vi "Keyence.FTP.GetLastFile.vi"(5 "Bank (0)":u8, 7 "LogPath":path=path "C:/SOFTWARE/logs/scanner", 8 "error in (no error)":errorcluster, 11 "FTP Session out":T1) -> (0 "error out":errorcluster, 3 "File name":path)   [LabVIEW 2016]
uses:
  <vilib>/FTP/ftp0.llb/FTP Session.ctl
  <vilib>/FTP/NI_FTP.lvlib
panel:
  out "Files":string[](array[string])
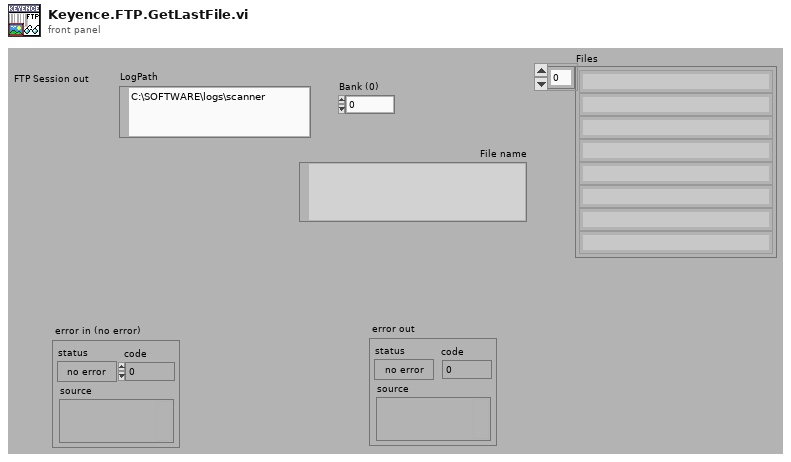
[diagram p1: front panel]
types:
  T1 = typedef "NI_FTP.lvlib/FTP Session.ctl" = refnum<k5>
  T2 = typedef "NI_FTP.lvlib/FTP File Info.ctl" = cluster{"type":enum16{"unknown", "file", "dir", "link"}, "permissions":string, "owner":string, "group":string, "size":i32, "date":string, "name":string, "link name":string}
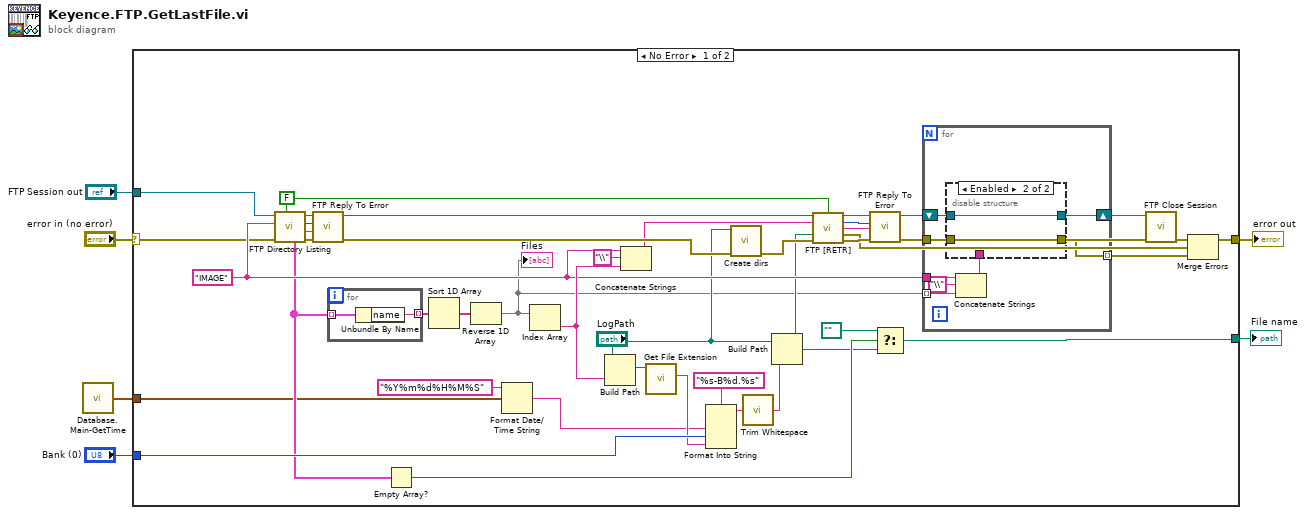
[diagram p0: block diagram]
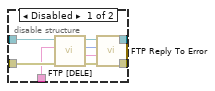
[diagram p2: hidden frame]
diagram:
  n1 = call "Database.Main-GetTime.vi"() -> ("TS"=w1:timestamp)  [unwired: 1 in]
  n2 = case shown="No Error" "error in (no error)" {
    selector: "error in (no error)" -> [w10 w71]
    tunnel: [w35 w71] -> w6
    tunnel: [w14 _] -> w4
    tunnel: "Bank (0)" -> [w25 _]
    tunnel: "FTP Session out" -> [w11 _]
    tunnel: w1 -> [w7 _]
    frame No Error {
      w19 = "IMAGE" ("directory path")
      w43 = FALSE ("active (T)")
      n3 = call <vilib>:"FTP Directory Listing.vi"("active (T)"=w43, "error in (no error)"=w10, "directory path"=w19, "ftp session"=w11) -> ("error out"=w47:errorcluster, "reply string"=w45:string, "reply code"=w46:i32, "ftp session out"=w48:T1, "dir list"=w17:T2[])  [unwired: 3 in]
      n4 = call <vilib>:"FTP Reply To Error.vi"("error in (no error)"=w47, "reply string in"=w45, "reply code in"=w46, "ftp session"=w48) -> ("error out"=w28:errorcluster, "ftp session out"=w44:T1)  [unwired: 2 out]
      n5 = for {
        tunnel: w17 -> [w51] mode=indexing
        tunnel: [w50] -> w22 mode=indexing
        n6 = Unbundle By Name(w51) -> ("name"=w50:string)
      }
      n7 = Empty Array?(array=w17) -> (empty?=w16:bool)
      n8 = Sort 1D Array(array=w22) -> (sorted array=w21:string[])
      n9 = Reverse 1D Array(array=w21) -> (reversed array=w12:string[])
      "Files" <- w12
      n10 = Format Date/Time String(time format string (%c)="%Y%m%d%H%M%S", seconds (now)=w7) -> (date/time string=w8:string)  [unwired: 1 in]
      n11 = Index Array(array=w12) -> (element=w20:string)  [unwired: 1 in]
      n12 = Build Path(base path="LogPath", name or relative path=w20) -> (appended path=w38:path)
      n13 = Concatenate Strings(w19, "\\" ("string"), w20) -> (w23:string)
      n14 = call <vilib>:"Get File Extension.vi"("file"=w38) -> ("lowercase file extension"=w24:string)  [unwired: 6 in, 4 out]
      n15 = Format Into String(format string="%s-B%d.%s", w8, w25, w24) -> (resulting string=w37:string)  [unwired: 2 in, 1 out]
      n16 = call "Create dirs.vi"("error in (no error)"=w28, "deepest dir"="LogPath") -> ("error"=w27:errorcluster)  [unwired: 9 in]
      n17 = call <vilib>:"Trim Whitespace.vi"("string"=w37) -> ("trimmed string"=w34:string)  [unwired: 1 in]
      n18 = Build Path(base path="LogPath", name or relative path=w34) -> (appended path=w15:path)
      n19 = call <vilib>:"FTP [RETR].vi"("ftp session"=w44, "active (T)"=w43, "remote path"=w23, "local path (<NAP>)"=w15, "error in (no error)"=w27) -> ("ftp session out"=w42:T1, "reply code"=w40:i32, "reply string"=w39:string, "file error"=w36:errorcluster, "error out"=w41:errorcluster)  [unwired: 1 in, 5 out]
      n20 = call <vilib>:"FTP Reply To Error.vi"("error in (no error)"=w41, "reply string in"=w39, "reply code in"=w40, "ftp session"=w42) -> ("error out"=w33:errorcluster, "ftp session out"=w32:T1)  [unwired: 2 out]
      n21 = Select(t=path "", s=w16, f=w15) -> (s? t:f=w14:path)
      n22 = for {
        tunnel: w33 -> [w59]
        tunnel: w12 -> [w52] mode=indexing
        tunnel: w19 -> [w57]
        tunnel: [w54] -> w31 mode=indexing
        shift-right: [w53] -> w30
        shift-left: w32 -> [w58]
        n23 = Concatenate Strings(w57, "\\" ("string"), w52) -> (w56:string)
        n24 = disable-structure shown="Enabled" {
          disable-tunnel: w59 -> [w68 w69]
          disable-tunnel: w58 -> [w67 w70]
          disable-tunnel: w56 -> [w62 _]
          disable-tunnel: [w61 w69] -> w54
          disable-tunnel: [w60 w70] -> w53
          frame Disabled {
            n25 = call <vilib>:"FTP [DELE].vi"("error in (no error)"=w68, "file path"=w62, "ftp session"=w67) -> ("error out"=w66:errorcluster, "reply string"=w63:string, "reply code"=w64:i32, "ftp session out"=w65:T1)  [unwired: 5 in]
            n26 = call <vilib>:"FTP Reply To Error.vi"("error in (no error)"=w66, "reply string in"=w63, "reply code in"=w64, "ftp session"=w65) -> ("error out"=w61:errorcluster, "ftp session out"=w60:T1)  [unwired: 2 out]
          }
          frame Enabled {
          }
        }
      }
      n27 = call <vilib>:"FTP Close Session.vi"("error in (no error)"=w33, "ftp session"=w30) -> ("error out"=w49:errorcluster)  [unwired: 6 in, 3 out]
      n28 = Merge Errors(w49, w36, w31) -> (w35:errorcluster)
    }
    frame Error {
    }
  }
  "error out" <- w6
  "File name" <- w4
